vi "Read owner.vi"(8 "error in (no error)":errorcluster, 11 "Product-A in":refnum<class "Product-A.lvclass">) -> (0 "error out":errorcluster, 2 "owner":string, 3 "Product-A out":refnum<class "Product-A.lvclass">)   [LabVIEW 2018, in "Product-A.lvclass"]
uses:
  Product-A.lvclass
  Product-A.lvclass/Product-A.ctl
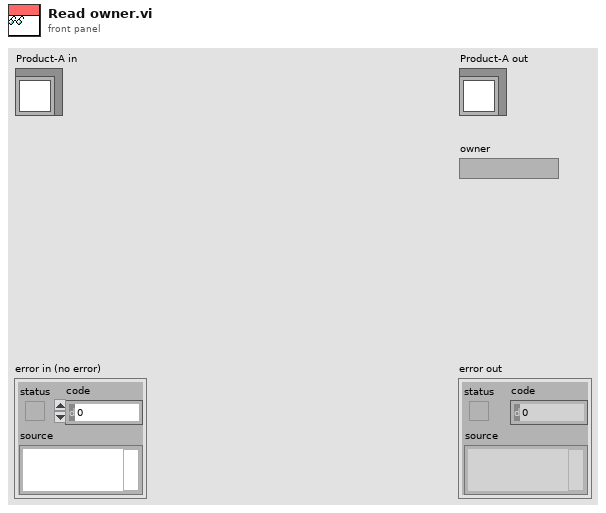
[diagram p1: front panel]
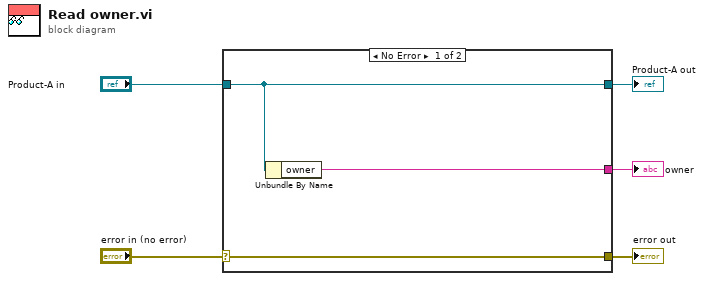
[diagram p0: block diagram]
diagram:
  n1 = case shown="No Error" "error in (no error)" {
    selector: "error in (no error)" -> [w8 w9]
    tunnel: [w8 w9] -> w4
    tunnel: [w7 w10] -> w2
    tunnel: "Product-A in" -> [w7 w10]
    tunnel: [w6 _] -> w1
    frame No Error {
      n2 = Unbundle By Name(w7) -> ("owner"=w6:string)
    }
    frame Error {
    }
  }
  "error out" <- w4
  "Product-A out" <- w2
  "owner" <- w1
